vi "TutorialGenAnalyzeDisp 2.vi"() -> ()   [LabVIEW 2012]
doc: "Use this template to generate a signal, analyze the signal, and display the result. You can use this template with the exercises in the Getting Started with LabVIEW manual.\nNote: LabVIEW enables automatic error handling by default for VIs you create from this template."
uses:
  Instance           1 34Saved   TutorialGenAnalyzeDisp.vit .vi
  Instance           2 34Saved   TutorialGenAnalyzeDisp.vit .vi
panel:
  out "Waveform Graph":dynamicdata(graph)
  out "RMS":dbl
  in  "stop":bool
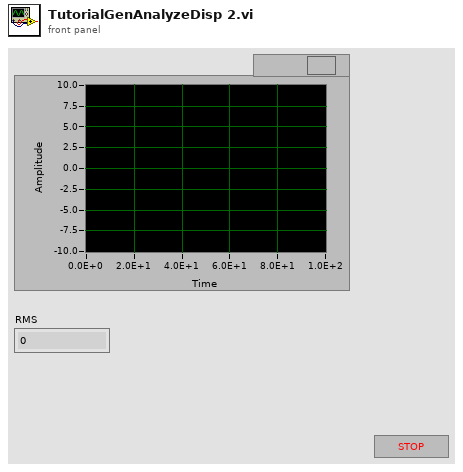
[diagram p1: front panel]
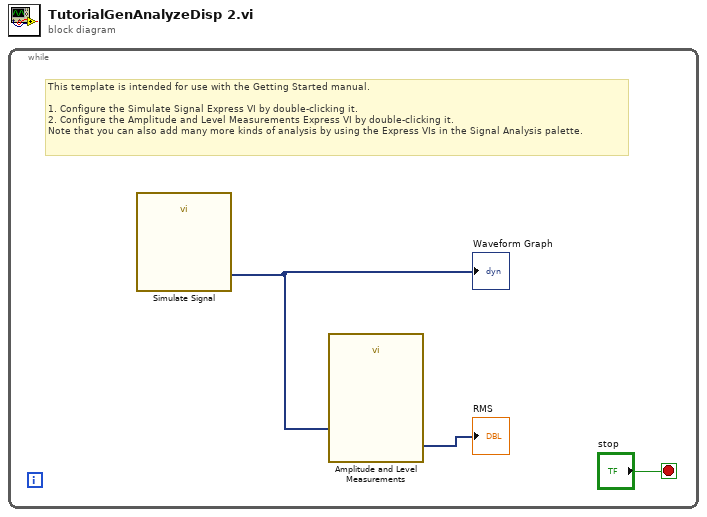
[diagram p0: block diagram]
diagram:
  n1 = while {
    stop <- "stop" stop-if-true
    # "This template is intended for use with the Getting Started manual.\n\n1. Configure the Simulate Signal Express VI by double-clicking it.\n2. Configure the Amplitude and Level Measurements Express VI by double-clicking it.\nNote that you can also add many more kinds of analysis by using the Express VIs in the Signal Analysis palette."
    n2 = call "Simulate Signal"() -> ("Sine"=w2:dynamicdata)  [unwired: 14 in, 1 out]
    "Waveform Graph" <- w2
    n3 = call "Amplitude and Level Measurements"("Signals"=w2) -> ("RMS"=→"RMS":dynamicdata)  [unwired: 13 in, 1 out]
  }
